vi "GL_Modulo_Triggers.vi"(0 "GL Ref In":refnum<k7>, 1 "Axis":u16(ring)=1 items=["Axis 1"=1, "Axis 2"=2, "Axis 3"=3, "Axis 4"=4, "Axis 5"=5, "Axis 6"=6, "Axis 7"=7, "Axis 8"=8], 2 "Reverse ?":bool, 5 "Program Name":string caption="Beginning Text", 7 "Motion Settings In":T1={"No Motion?"=FALSE, "Motion System"=enum."NI 735x", "Motion Bd ID"=1, "Motion Profile"="SMAC1", "# Axis"=1, "Reverse Z axis?"=TRUE, "SMAC Axis"=0, "scan pair"=enum."y-(x) scan", "RT fps"=6.0, "Steps per mm"=[1000, 1000, 1000, 1000], "Motor Parameters"={"velocity ct/s"=[10000.0, 10000.0, 10000.0, 50000.0], "accel ct/s^2"=[50000.0, 50000.0, 50000.0, 200000.0]}, "One Way Scan"=FALSE, "Reverse One Way Scan"=FALSE, "Global Position (mm)"=[], "Plane"=0, "Distance between\nscan lines (um)"=0.0, "Distance between\nscan planes (um)"=0.0, "number of scan planes"=1, "Total steps in line"=0, "Xtra plane\ndistance  (um)"=100, "Xtra planes "=1, "Add Axis"=FALSE, "overshoot cts"=200, "BKPT Shift"=0, "Scan Start Time (ms)"=0, "ESP VISA"="GPIB::1::INSTR", "3rd Axis"=1, "GL Ref Out"=refnum, "Galil Address"=""} {"3rd Axis" items=["x", "y", "z", "w"]; "Xtra planes" min=1; "Xtra plane\ndistance  (um)" min=0; "Distance between\nscan planes (um)" format="%.2f"; "Distance between\nscan lines (um)" format="%.2f"; "SMAC Axis" items=["None"=0, "Axis 1"=1, "Axis 2"=2, "Axis 3"=3, "Axis 4"=4, "Axis 5"=5, "Axis 6"=6, "Axis 7"=7, "Axis 8"=8, "Vector Space 1"=17, "Vector Space 2"=18, "Vector Space 3"=19, "Vector Space 4"=20]; "Motion Bd ID" min=1 max=32 step=1}, 11 "error in":errorcluster, 13 "Start Position":i32) -> (4 "GL Ref Out":refnum<k7>, 6 "Axis Out":u16(ring)=1 items=["Axis 1"=1, "Axis 2"=2, "Axis 3"=3, "Axis 4"=4, "Axis 5"=5, "Axis 6"=6, "Axis 7"=7, "Axis 8"=8], 15 "error out":errorcluster)   [LabVIEW 2022 SP3]
doc: "EXAMPLE: DO_WHILE Loop (Onboard Programming Template)\n\nSUMMARY:\nThis FlexMotion example demonstrates the implementation of a DO_WHILE loop data structure in an onboard program. The C equivalent of the data structure implemented here is:\n\ndo {\n// code to be repeated\nloopVar = loopVar - increment;\n} while (loopVar != 0);\n\nTHEORY OF OPERATION:\nThe flow of the DO_WHILE loop data structure goes as follows:\n(1) Program storage is begun.\n(2) The DO_WHILE loop is set up. (Loop Variable and Increment are each defined and initialized.)\n(3) A code delimiter is set using label #1.\n(4) Code to be executed each time through loop is run (in the template program, the loop variable is decremented).\n(5) The loop variable or other test condition is checked.\n(6) If the test condition is true, then we jump back to label #1. Otherwise, the condition is false so the loop terminates.\n(7) Program storage is ended.\n\nDEVELOPMENT DETAILS:\nApplication Software: LabVIEW 5.0.x\nHardware: FlexMotion controller\nDriver Software: FlexMotion Software 4.0\n\nREQUIRED HARDWARE:\n(controller only)\n\nINSTRUCTIONS:\n(0) Initialize the FlexMotion controller before running this VI. \n(1) Add the FlexMotion functions you want to execute into the block diagram where noted.\n(2) Run the VI to store the program. (The program will not be executed at this time.)\n(3) You can then run the program you have stored by calling the run_prog.flx function with the appropriate program number.\n\nADDITIONAL NOTES:\n(a) You should read the following items before writing FlexMotion onboard programs:\n(1) The Onboard Programs section of the FlexMotion Hardware User Manual (page 4-9 in the November 1998 edition).\n(2) The section about onboard variables in your FlexMotion Software Reference Manual (pages 4-11 and 4-12 in the November 1998 edition)\n(3) You will find the chapter of the FlexMotion Software Reference Manual concerning the Onboard Programming functions to be an invaluable reference resource (Chapter 12 of the November 1998 edition) along with the online help for the VI functions.\n(b) This template repeats the DO_WHILE loop as long as an expression with a variable evaluates to be true. However, you may evaluate other conditions such as move complete status instead.\n\n*NOTE: This example is not supported on the 7334 controller."
uses:
  NI_controller/-NI_MotionRoutines/MotionParameters.ctl
  NI_controller/-NI_MotionRoutines/MotionSys.ctl
  -MotionRoutines/ScanAxis.ctl
  -MotionRoutines/3rdAxis.ctl
panel:
  # "1-D and 2-D B scan settings"
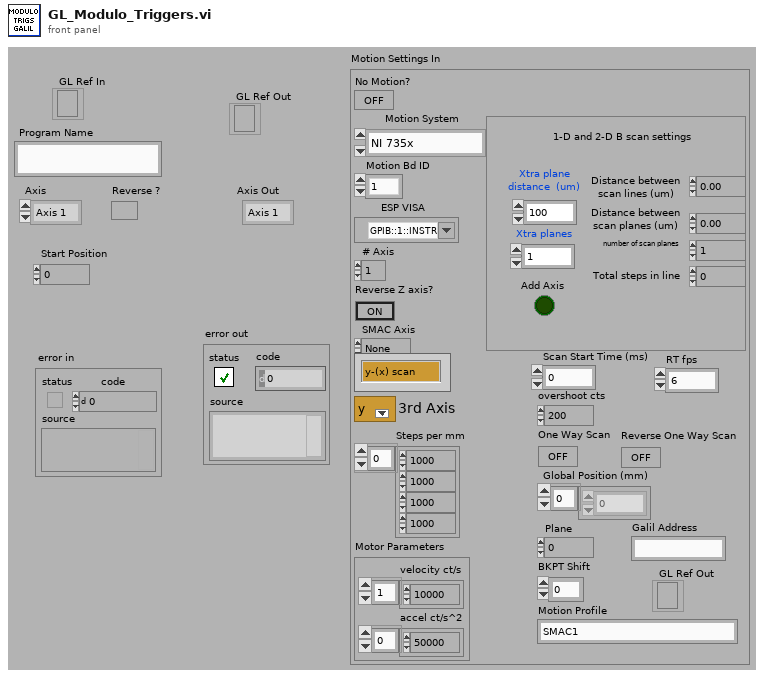
[diagram p1: front panel]
types:
  T1 = typedef "MotionParameters.ctl" = cluster{"No Motion?":bool, "Motion System":T2, "Motion Bd ID":u8, "Motion Profile":string, "# Axis":i8, "Reverse Z axis?":bool, "SMAC Axis":u16, "scan pair":T3, "RT fps":sgl, "Steps per mm":i32[], "Motor Parameters":cluster{"velocity ct/s":dbl[], "accel ct/s^2":dbl[]}, "One Way Scan":bool, "Reverse One Way Scan":bool, "Global Position (mm)":dbl[], "Plane":i32, "Distance between\nscan lines (um)":sgl, "Distance between\nscan planes (um)":sgl, "number of scan planes":i32, "Total steps in line":i32, "Xtra plane\ndistance  (um)":i32, "Xtra planes ":i32, "Add Axis":bool, "overshoot cts":i32, "BKPT Shift":i32, "Scan Start Time (ms)":u32, "ESP VISA":refnum<visa-resource-name>, "3rd Axis":T4, "GL Ref Out":refnum<k7>, "Galil Address":string}
  T2 = typedef "MotionSys.ctl" = enum16{"MM3000", "NI 735x", "Newport ESP", "No Motion Card", "Galil"}
  T3 = typedef "ScanAxis.ctl" = enum16{"y-(x) scan", "x-(y) scan", "z-(x) scan", "z-(y) scan", "y-(z) scan", "x-(z) scan", "w-(x) scan", "w-(y) scan", "w-(z) scan", "x-(w) scan", "y-(w) scan", "z-(w) scan"}
  T4 = typedef "3rdAxis.ctl" = u16
  T5 = enum16{"Less Than", "Equal", "Less Than Or Equal", "Greater Than", "Not Equal", "Greater Than Or Equal", "True", "Home Found", "Index Found", "High Speed Capture", "Position Breakpoint", "Reserved", "Velocity Threshold", "Move Complete", "Profile Complete", "Blend Complete", "Motor Off", "Home Input Active", "Limit Input Active", "Software Limit Active", "Program Complete", "IO Port Match"}
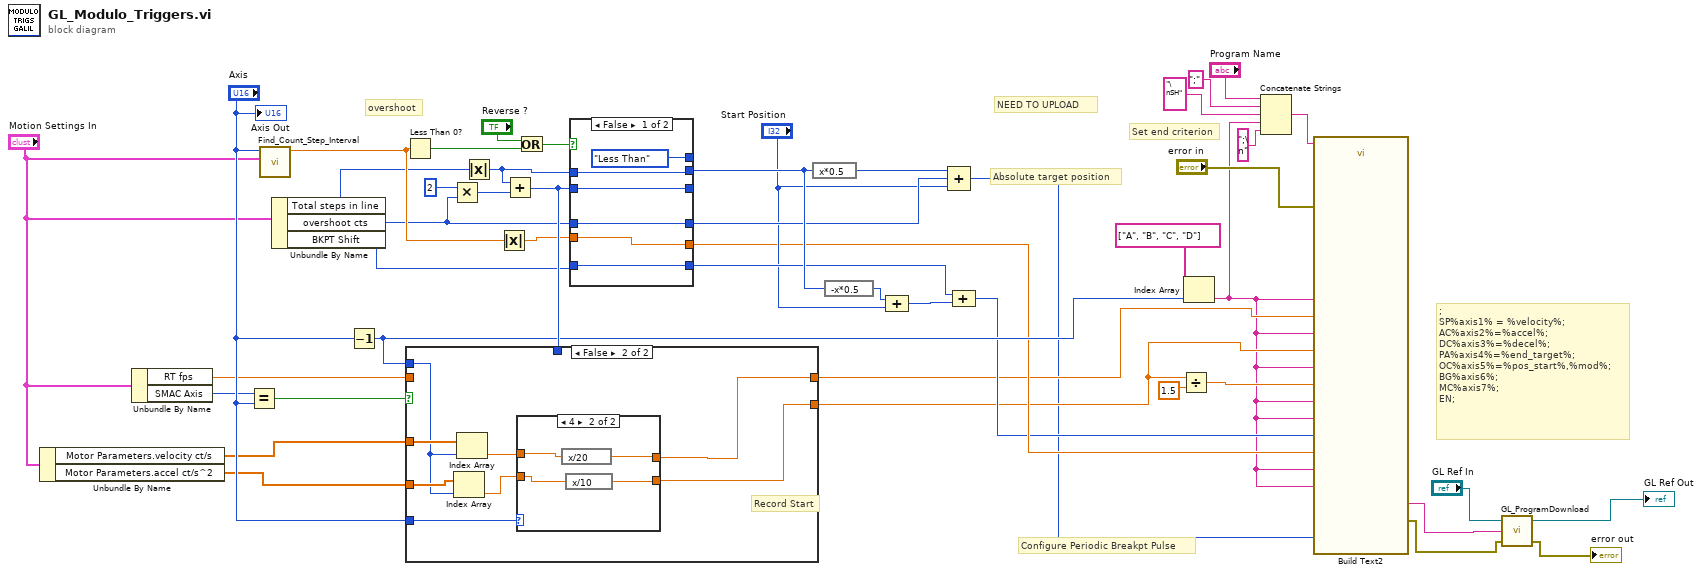
[diagram p0: block diagram]
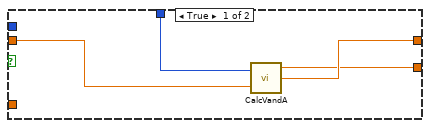
[diagram p2: hidden frame]
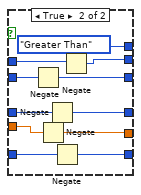
[diagram p4: hidden frame]
diagram:
  # "NEED TO UPLOAD"
  # ";\nSP%axis1% = %velocity%;\nAC%axis2%=%accel%;\nDC%axis3%=%decel%;\nPA%axis4%=%end_target%;\nOC%axis5%=%pos_start%,%mod%;\nBG%axis6%;\nMC%axis7%;\nEN;"
  # "Absolute target position"
  # "Configure Periodic Breakpt Pulse"
  # "Set end criterion"
  # "overshoot"
  # "Record Start"
  n1 = Unbundle By Name("Motion Settings In") -> ("Motor Parameters.velocity ct/s"=w21:dbl[], "Motor Parameters.accel ct/s^2"=w22:dbl[])
  n2 = Unbundle By Name("Motion Settings In") -> ("RT fps"=w29:sgl, "SMAC Axis"=w31:u16)
  n3 = Equal?(x=w31, y="Axis") -> (x = y?=w26:bool)
  n4 = call "Find_Count_Step_Interval.vi"("Motion Settings In"="Motion Settings In", "Axis"="Axis") -> ("BP Interval"=w33:dbl)  [unwired: 8 in, 1 out]
  n5 = Unbundle By Name("Motion Settings In") -> ("Total steps in line"=w28:i32, "overshoot cts"=w23:i32, "BKPT Shift"=w19:i32)
  n6 = Decrement(x="Axis") -> (x-1=w20:u16)
  n7 = Less Than 0?(x=w33) -> (x < 0?=w47:bool)
  n8 = Multiply(x=2, y=w23) -> (x*y=w42:i32)
  n9 = Absolute Value(x=w28) -> (abs(x)=w44:i32)
  n10 = Absolute Value(x=w33) -> (abs(x)=w27:dbl)
  n11 = Add(x=w44, y=w42) -> (x+y=w41:i32)
  n12 = case shown="False" w26 {
    tunnel: [w48 w59] -> w15
    tunnel: [w49 w57] -> w14
    tunnel: w41 -> [w51 _]
    tunnel: w29 -> [w50 _]
    tunnel: "Axis" -> [_ w58]
    tunnel: w22 -> [_ w56]
    tunnel: w20 -> [_ w52]
    tunnel: w21 -> [_ w55]
    frame True {
      n13 = call "CalcVandA.vi"("distance"=w51, "fps"=w50) -> ("Accel"=w48:dbl, "Velocity"=w49:dbl)  [unwired: 1 out]
    }
    frame False {
      n14 = Index Array(array=w56, index=w52) -> (element=w53:dbl)
      n15 = Index Array(array=w55, index=w52) -> (element=w54:dbl)
      n16 = case shown="4" w58 {
        tunnel: w54 -> [w61 w65]
        tunnel: w53 -> [w60 w62]
        tunnel: [w61 w64] -> w57
        tunnel: [w60 w63] -> w59
        frame 0, Default {
        }
        frame 4 {
          n17 = expression code="x/20"(w65) -> (w64:dbl)
          n18 = expression code="x/10"(w62) -> (w63:dbl)
        }
      }
    }
  }
  n19 = Or(x="Reverse ?", y=w47) -> (x .or. y?=w45:bool)
  n20 = case shown="False" w45 {
    tunnel: w41 -> [w71 w82]
    tunnel: [w71 w81] -> _
    tunnel: [T5."Less Than" ("Condition Code (True)") T5."Greater Than" ("Condition Code (True)")] -> _
    tunnel: [w69 w78] -> w38
    tunnel: w23 -> [w69 w79]
    tunnel: w27 -> [w68 w77]
    tunnel: [w68 w76] -> w18
    tunnel: [w67 w74] -> w40
    tunnel: w44 -> [w67 w75]
    tunnel: w19 -> [w66 w73]
    tunnel: [w66 w72] -> w34
    frame False {
    }
    frame True {
      n21 = Negate(x=w82) -> (-x=w81:i32)
      n22 = Negate(x=w77) -> (-x=w76:dbl)
      n23 = Negate(x=w79) -> (-x=w78:i32)
      n24 = Negate(x=w73) -> (-x=w72:i32)
      n25 = Negate(x=w75) -> (-x=w74:i32)
    }
  }
  n26 = expression code="x*0.5"(w40) -> (w39:i32)
  n27 = expression code="-x*0.5"(w40) -> (w36:i32)
  n28 = Compound Arithmetic op=ADD(w36, "Start Position") -> (w35:i32)
  n29 = Compound Arithmetic op=ADD(w39, w38, "Start Position") -> (w12:i32)
  n30 = Compound Arithmetic op=ADD(w34, w35) -> (w17:i32)
  n31 = Divide(x=w15, y=1.5) -> (x/y=w16:dbl)
  n32 = Index Array(array=string[] ["A", "B", "C", "D"], index=w20) -> (element=w5:string)
  n33 = Concatenate Strings("Program Name", ";", "\nSH", w5, ";\n") -> (w4:string)
  n34 = call "Build Text2"("Beginning Text"=w4, "axis1"=w5, "velocity"=w14, "axis2"=w5, "accel"=w15, "axis3"=w5, "decel"=w16, "error in (no error)"="error in", "axis4"=w5, "end_target"=w12, "axis5"=w5, "pos_start"=w17, "mod"=w18, "axis6"=w5, "axis7"=w5) -> ("Result"=w8:string, "error out"=w9:errorcluster)  [unwired: 11 in]
  n35 = call "GL_ProgramDownload.vi"("error in"=w9, "program"=w8, "Galil.IGalil"="GL Ref In") -> ("error out"=→"error out":errorcluster, "reference out"=→"GL Ref Out":refnum<k7>)  [unwired: 1 out]
  "Axis Out" <- "Axis"
